vi "XL320_Read Motor Velocity.vi"(8 "error in (no error)":errorcluster, 10 "Motor ID (0)":u8, 11 "VISA resource name":refnum<visa-resource-name>) -> (0 "error out":errorcluster, 2 "Velocity (RPM)":dbl, 3 "VISA resource name out":refnum<visa-resource-name>)   [LabVIEW 2017, in "Dynamixel XL320.lvlib"]
doc: "Retrieves the motor's velocity."
uses:
  <instrlib>/Dynamixel XL320 (Drivers instrument)/Dynamixel XL320.lvlib
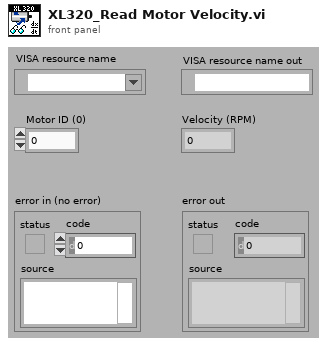
[diagram p1: front panel]
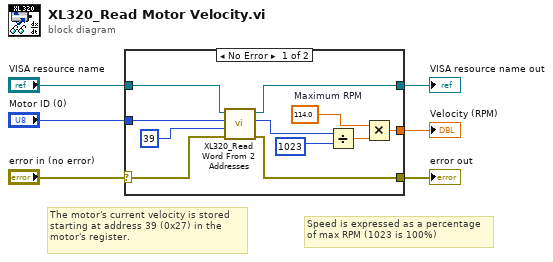
[diagram p0: block diagram]
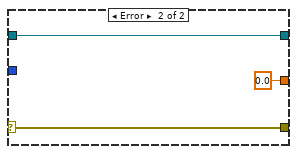
[diagram p2: hidden frame]
diagram:
  # "The motor's current velocity is stored\nstarting at address 39 (0x27) in the\nmotor's register."
  # "Speed is expressed as a percentage \nof max RPM (1023 is 100%)"
  n1 = case shown="No Error" "error in (no error)" {
    selector: "error in (no error)" -> [w10 w19]
    tunnel: "VISA resource name" -> [w13 w20]
    tunnel: [w9 w20] -> w5
    tunnel: [w7 w19] -> w4
    tunnel: [w15 0.0] -> w3
    tunnel: "Motor ID (0)" -> [w12 _]
    frame No Error {
      w14 = 114.0  # Maximum RPM
      n2 = call <instrlib>:"XL320_Read Word From 2 Addresses.vi"("Error in (no error)"=w10, "Address number (0)"=u16 39 ("Address # DEC"), "Motor ID (0)"=w12, "VISA resource name"=w13) -> ("error out"=w7:errorcluster, "Data"=w8:u16, "VISA resource name out"=w9:refnum<visa-resource-name>)  [unwired: 5 in]
      n3 = Divide(x=w8, y=1023) -> (x/y=w16:dbl)
      n4 = Multiply(x=w14, y=w16) -> (x*y=w15:dbl)
    }
    frame Error {
    }
  }
  "VISA resource name out" <- w5
  "error out" <- w4
  "Velocity (RPM)" <- w3
